vi "Csengő.vi"() -> ()   [LabVIEW 2014]
doc: "Az alkalmazás képes egy iskolai csengõ szerepét betölteni, csengetés hangot lejátszva a szükséges idõpontokban, figyelembe véve az aktuális tanév rendjét(ezt minden tanévben egyszer be kell állítani). Ezentúl beállítható, hogy a rendes, vagy a rövidített csengetési rend legyen érvényes egy adott napon. A szoftverben továbbá beállíthatóak olyan napok, mikor csak az elsõ n óra van megtartva. Segítségével egyszerûen, olcsón, az iskolarádióval egybevonva üzemeltethetõ az iskolacsengõ. A szoftver ezek mellett tûzriadó és bombariadó esetén képes riadójelzést sugározni.\n\nA mûködéssel kapcsolatos bõvebb információkért nyissa meg az alkalmazáson belül is megnyitható, az alkalmazás saját \"Olvass el!\" fájlát."
uses:
  <vilib>/Utility/file.llb/Read From Spreadsheet File (string).vi
  <vilib>/Utility/file.llb/Write To Spreadsheet File (string).vi
panel:
  out "Tanítási nap":bool
  in  "Segítség":bool
  out "Speciális tanítás":bool
  in  "Leállítás":bool
  in  "Módosítás":bool
  out "Kevesebb tanóra":bool
  out "Jelzõcsengõ":bool
  out "Csengõ":bool
  out "Munkaszüneti nap/\nSzünet":bool
  out "Napi max\nÓraszám:":i32
  out "Csengetési rend":string[][](array[string])
  out "Szünetek":string[][](array[string])
  out "Rövidített óra led":bool
  in  "Rövidített óra":bool
  out "Bombariadó LED":bool
  out "Tûzriadó LED":bool
  in  "Bombariadó":bool
  in  "Tûzriadó":bool
  # "Manuális vezérlés:"
  # "Tantervek módosítása"
  # "Táblázatok:"
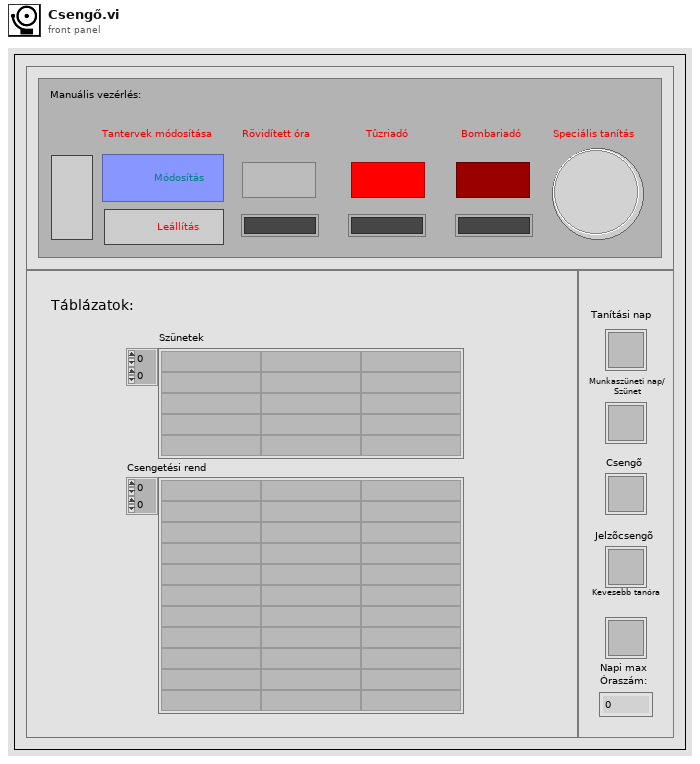
[diagram p1: front panel]
types:
  T1 = enum16{"open", "replace", "create", "open or create", "replace or create", "replace or create with confirmation"}
  T2 = typedef "LVDateTimeRec.ctl" = cluster{"fractional second":dbl, "second":i32, "minute":i32, "hour":i32, "day of month":i32, "month":i32, "year":i32, "day of week":i32, "day of year":i32, "DST":i32}
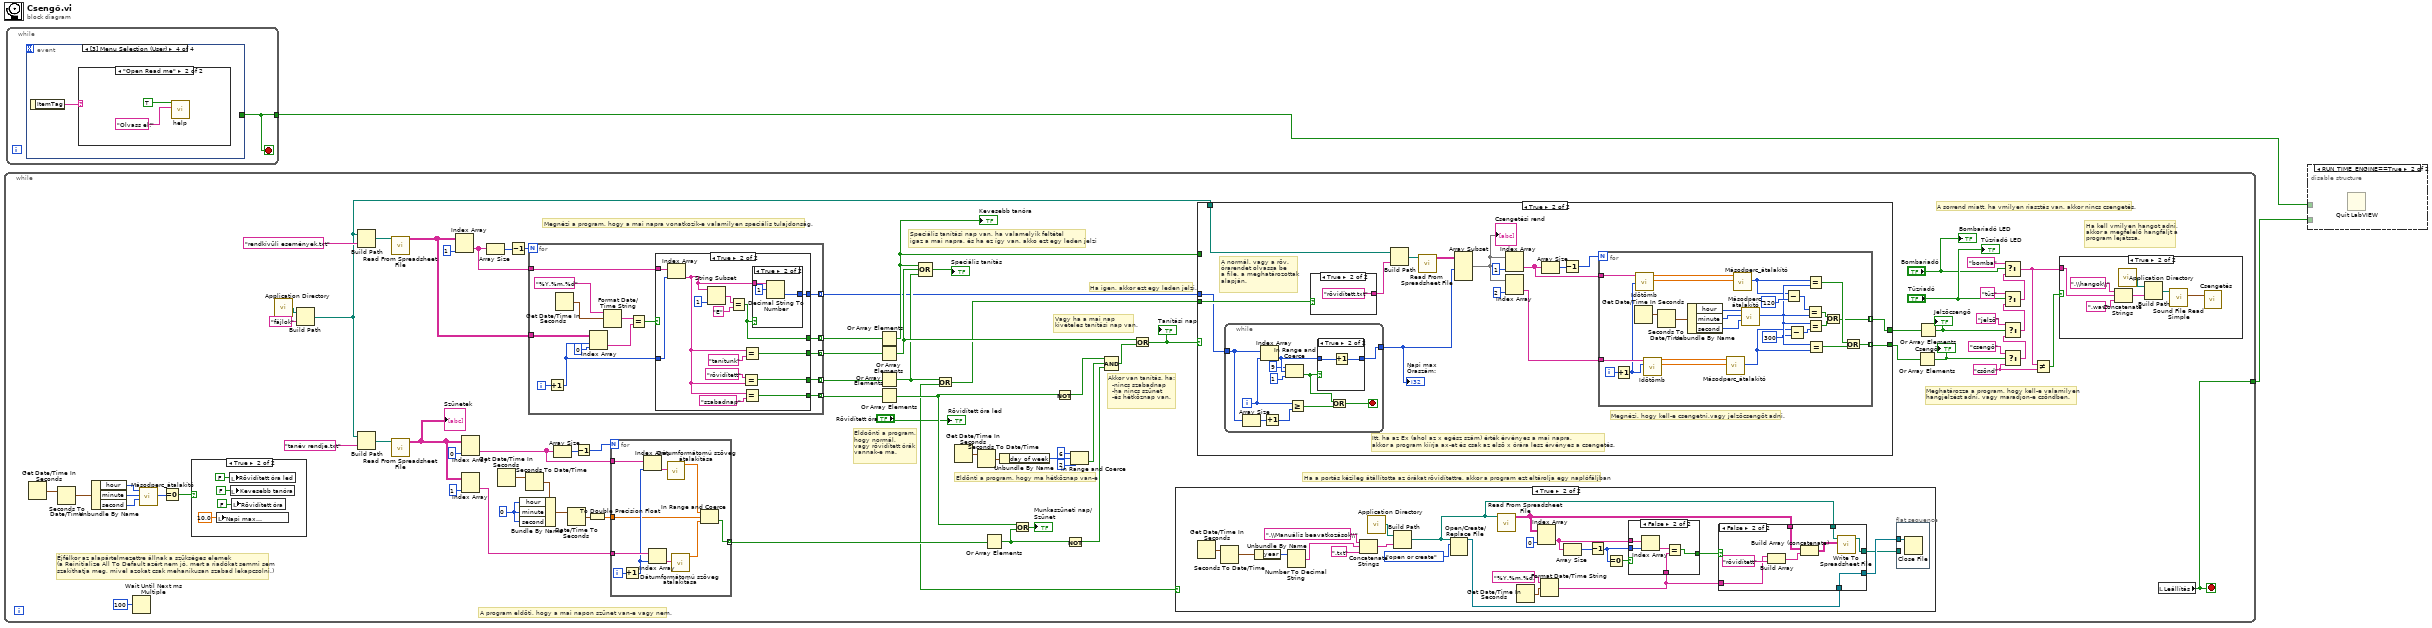
[diagram p0: block diagram]
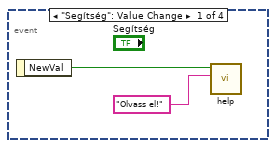
[diagram p3: hidden frame]
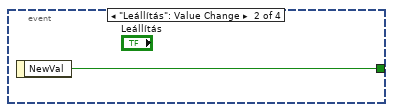
[diagram p4: hidden frame]
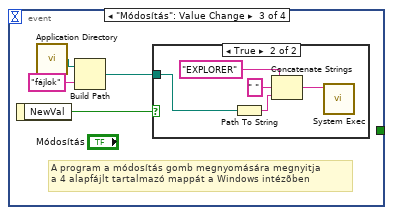
[diagram p5: hidden frame]
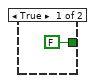
[diagram p11: hidden frame]
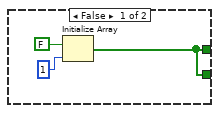
[diagram p13: hidden frame]
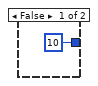
[diagram p14: hidden frame]
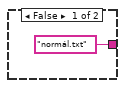
[diagram p15: hidden frame]
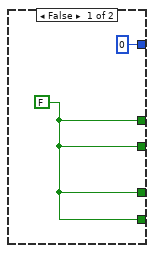
[diagram p16: hidden frame]
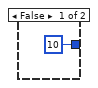
[diagram p17: hidden frame]
diagram:
  n1 = while {
    tunnel: [w3] -> w2
    stop <- w3 stop-if-true
    w36 = "csönd" ("format string")
    w61 = 0 ("hour")
    # "A sorrend miatt, ha vmilyen riasztás van, akkor nincs csengetés."
    # "Ha kell vmilyen hangot adni,\nakkor a megfelelõ hangfáljt a\nprogram lejátsza."
    # "Meghatározza a program, hogy kell-e valamilyen\nhangjelzést adni, vagy maradjon-e csöndben."
    # "Eldoönti a program,\nhogy normál,\nvagy rövidített órák\nvannak-e ma."
    # "Speciális tanítási nap van, ha valamelyik feltétel\nigaz a mai napra, és ha ez így van, akko ezt egy leden jelzi"
    # "Ha igen, akkor ezt egy leden jelzi."
    # "Eldönti a program, hogy ma hétköznap van-e"
    # "Vagy ha a mai nap\nkivételes tanítási nap van."
    # "Akkor van tanítás, ha:\n  -nincs szabadnap\n  -ha nincs szünet\n  -és hétköznap van."
    # "A program eldöti, hogy a mai napon szünet van-e vagy nem."
    # "Megnézi a program, hogy a mai napra vonatkozik-e valamilyen speciális tulajdonság."
    # "Ha a portás kézileg átállította az órákat rövidítettre, akkor a program ezt eltárolja egy naplófáljban"
    # "Éjfélkor az alapártelmezettre állnak a szükséges elemek\n(a Reinitialize All To Default azért nem jó, mert a riadókat semmi sem\nszakíthatja meg, mivel azokat csak mehanikusan szabad lekapcsolni.)"
    n2 = Get Date/Time In Seconds() -> (seconds since 1Jan1904=w13:timestamp)
    n3 = Seconds To Date/Time(time stamp (now)=w13) -> (date time rec=w12:T2)  [unwired: 1 in]
    n4 = Unbundle By Name(w12) -> ("hour"=w11:i32, "minute"=w10:i32, "second"=w9:i32)
    n5 = Wait Until Next ms Multiple(millisecond multiple=u32 100) -> ()  [unwired: 1 out]
    n6 = call "Másodperc_átalakító.vi"("Másodperc érték"=w9, "Perc érték"=w10, "Óra érték"=w11) -> ("Az összes érték másodpercben"=w14:i32)  [unwired: 8 in]
    n7 = Equal To 0?(x=w14) -> (x = 0?=w8:bool)
    n8 = case shown="True" w8 {
      frame False {
      }
      frame True {
        n9 = local write "Napi max\nÓraszám:"(10.0 ("Óraszám:")) -> ()
        n10 = local write "Rövidített óra led"(FALSE ("Rövidített óra led")) -> ()
        n11 = local write "Kevesebb tanóra"(FALSE ("Kevesebb tanóra")) -> ()
        n12 = local write "Rövidített óra"(FALSE ("Rövidített óra")) -> ()
      }
    }
    n13 = call <vilib>:"Application Directory.vi"() -> ("Application Directory"=w77:path)
    n14 = Build Path(base path=w77, name or relative path="fájlok") -> (appended path=w7:path)
    n15 = Build Path(base path=w7, name or relative path="rendkívüli események.txt") -> (appended path=w71:path)
    n16 = Build Path(base path=w7, name or relative path="tanév rendje.txt") -> (appended path=w69:path)
    n17 = call-poly <vilib>:"Read From Spreadsheet File.vi"("file path (dialog if empty)"=w71) -> ("all rows"=w49:string[][])  [unwired: 6 in, 4 out]
    n18 = call-poly <vilib>:"Read From Spreadsheet File.vi"("file path (dialog if empty)"=w69) -> ("all rows"=w41:string[][])  [unwired: 6 in, 4 out]
    "Szünetek" <- w41
    n19 = Index Array(array=w49, index (col)=1 ("index (row)")) -> (element=w50:string[])  [unwired: 1 in]
    n20 = Index Array(array=w41, index (col)=0 ("disabled index (col)")) -> (element=w57:string[])  [unwired: 1 in]
    n21 = Index Array(array=w41, index (col)=1 ("disabled index (col)")) -> (element=w53:string[])  [unwired: 1 in]
    n22 = Array Size(array=w50) -> (size(s)=w74:i32)
    n23 = Get Date/Time In Seconds() -> (seconds since 1Jan1904=w63:timestamp)
    n24 = Decrement(x=w74) -> (x-1=w72:i32)
    n25 = Seconds To Date/Time(time stamp (now)=w63) -> (date time rec=w62:T2)  [unwired: 1 in]
    n26 = Bundle By Name(cluster=w62, "hour"=w61, "minute"=w61, "second"=w61) -> (w60:T2)
    n27 = for {
      N: w72 -> [_]
      tunnel: w50 -> [w206]
      tunnel: w49 -> [w210]
      tunnel: [w204] -> w46 mode=indexing
      tunnel: [w203] -> w48 mode=indexing
      tunnel: [w202] -> w47 mode=indexing
      tunnel: [w201] -> w45 mode=indexing
      tunnel: [w200] -> w26 mode=indexing
      i -> [w214]
      n28 = Increment(x=w214) -> (x+1=w205:i32)
      n29 = Get Date/Time In Seconds() -> (seconds since 1Jan1904=w213:timestamp)
      n30 = Index Array(array=w210, index (row)=w205, index (col)=0 ("disabled index (col)")) -> (element=w208:string)
      n31 = Format Date/Time String(time format string (%c)="%Y.%m.%d" ("format string"), seconds (now)=w213) -> (date/time string=w211:string)  [unwired: 1 in]
      n32 = Equal?(x=w211, y=w208) -> (x = y?=w207:bool)
      n33 = case shown="True" w207 {
        tunnel: w206 -> [_ w230]
        tunnel: w205 -> [_ w229]
        tunnel: [w216 w225] -> w204
        tunnel: [w216 w224] -> w203
        tunnel: [w216 w223] -> w202
        tunnel: [w216 w219] -> w201
        tunnel: [0 w217] -> w200
        frame False {
          w216 = FALSE
        }
        frame True {
          n34 = Index Array(array=w230, index=w229) -> (element=w218:string)
          n35 = String Subset(string=w218, length (rest)=1 ("length (rest)")) -> (substring=w220:string)  [unwired: 1 in]
          n36 = Equal?(x=w220, y="E") -> (x = y?=w219:bool)
          n37 = Equal?(x="rövidített", y=w218) -> (x = y?=w224:bool)
          n38 = Equal?(x=w218, y="tanítunk" ("x")) -> (x = y?=w225:bool)
          n39 = Equal?(x=w218, y="szabadnap" ("x")) -> (x = y?=w223:bool)
          n40 = case shown="True" w219 {
            tunnel: w218 -> [_ w234]
            tunnel: [10 w232] -> w217
            frame False {
            }
            frame True {
              n41 = Decimal String To Number(string=w234, offset=1) -> (number=w232:i32)  [unwired: 1 in, 1 out]
            }
          }
        }
      }
    }
    n42 = Array Size(array=w57) -> (size(s)=w54:i32)
    n43 = Date/Time To Seconds(2:w60) -> (0:w59:timestamp)  [unwired: 1 in]
    n44 = Decrement(x=w54) -> (x-1=w55:i32)
    n45 = To Double Precision Float(number=w59) -> (double precision float=w52:dbl)
    n46 = for {
      N: w55 -> [_]
      tunnel: w57 -> [w199]
      tunnel: w53 -> [w197]
      tunnel: w52 -> [w193]
      tunnel: [w190] -> w51 mode=indexing
      i -> [w198]
      n47 = Increment(x=w198) -> (x+1=w196:i32)
      n48 = Index Array(array=w199, index=w196) -> (element=w194:string)
      n49 = Index Array(array=w197, index=w196) -> (element=w195:string)
      n50 = call "Dátumformátomú szöveg átalakítása.vi"("Szöveg, amiben keresni kell"=w194) -> ("Dátum értéke számban"=w191:dbl)  [unwired: 10 in]
      n51 = call "Dátumformátomú szöveg átalakítása.vi"("Szöveg, amiben keresni kell"=w195) -> ("Dátum értéke számban"=w192:dbl)  [unwired: 10 in]
      n52 = In Range and Coerce(upper limit=w191, x=w193, lower limit=w192) -> (In Range?=w190:bool)  [unwired: 1 out]
    }
    n53 = Or Array Elements(Boolean array=w45) -> (logical OR=w27:bool)
    "Kevesebb tanóra" <- w27
    n54 = Or Array Elements(Boolean array=w46) -> (logical OR=w44:bool)
    n55 = Or Array Elements(Boolean array=w48) -> (logical OR=w43:bool)
    n56 = Or Array Elements(Boolean array=w47) -> (logical OR=w16:bool)
    n57 = Compound Arithmetic op=OR(w27, w44, w43) -> (→"Speciális tanítás":bool)
    n58 = Or(x=w43, y="Rövidített óra") -> (x .or. y?=w42:bool)
    n59 = Get Date/Time In Seconds() -> (seconds since 1Jan1904=w64:timestamp)
    n60 = Seconds To Date/Time(time stamp (now)=w64) -> (date time rec=w65:T2)  [unwired: 1 in]
    n61 = Or Array Elements(Boolean array=w51) -> (logical OR=w17:bool)
    n62 = Unbundle By Name(w65) -> ("day of week"=w66:i32)
    n63 = Or(x=w16, y=w17) -> (x .or. y?=→"Munkaszüneti nap/\nSzünet":bool)
    n64 = Not(x=w16) -> (.not. x?=w18:bool)
    n65 = Not(x=w17) -> (.not. x?=w19:bool)
    n66 = In Range and Coerce(upper limit=6, x=w66, lower limit=2) -> (In Range?=w20:bool)  [unwired: 1 out]
    n67 = Compound Arithmetic op=AND(w18, w20, w19) -> (w22:bool)
    n68 = Or(x=w44, y=w22) -> (x .or. y?=w21:bool)
    "Tanítási nap" <- w21
    n69 = case shown="True" "Rövidített óra" {
      frame False {
      }
      frame True {
        n70 = Get Date/Time In Seconds() -> (seconds since 1Jan1904=w90:timestamp)
        n71 = Seconds To Date/Time(time stamp (now)=w90) -> (date time rec=w89:T2)  [unwired: 1 in]
        n72 = Unbundle By Name(w89) -> ("year"=w88:i32)
        n73 = Number To Decimal String(number=w88) -> (decimal integer string=w86:string)  [unwired: 1 in]
        n74 = Concatenate Strings(".\\Manuális beavatkozások\\" ("string"), w86, ".txt" ("string")) -> (w93:string)
        n75 = call <vilib>:"Application Directory.vi"() -> ("Application Directory"=w92:path)
        n76 = Build Path(base path=w92, name or relative path=w93) -> (appended path=w85:path)
        n77 = Open/Create/Replace File(file path (use dialog)=w85, operation (0:open)=T1."open or create") -> (refnum out=w83:refnum<file>)  [unwired: 4 in, 2 out]
        n78 = call-poly <vilib>:"Read From Spreadsheet File.vi"("file path (dialog if empty)"=w85) -> ("all rows"=w98:string[][])  [unwired: 6 in, 4 out]
        n79 = Get Date/Time In Seconds() -> (seconds since 1Jan1904=w104:timestamp)
        n80 = Index Array(array=w98, index (col)=0 ("disabled index (col)")) -> (element=w99:string[])  [unwired: 1 in]
        n81 = Format Date/Time String(time format string (%c)="%Y.%m.%d." ("format string"), seconds (now)=w104) -> (date/time string=w97:string)  [unwired: 1 in]
        n82 = Array Size(array=w99) -> (size(s)=w96:i32)
        n83 = Decrement(x=w96) -> (x-1=w95:i32)
        n84 = Equal To 0?(x=w95) -> (x = 0?=w101:bool)
        n85 = case shown="False" w101 {
          tunnel: w99 -> [_ w121]
          tunnel: w95 -> [_ w120]
          tunnel: w97 -> [_ w118]
          tunnel: [FALSE w117] -> w100
          frame True {
          }
          frame False {
            n86 = Index Array(array=w121, index=w120) -> (element=w119:string)
            n87 = Equal?(x=w119, y=w118) -> (x = y?=w117:bool)
          }
        }
        n88 = case shown="False" w100 {
          tunnel: w98 -> [_ w114]
          tunnel: w85 -> [w106 w111]
          tunnel: w97 -> [_ w110]
          tunnel: [w107 w109] -> w84
          tunnel: w83 -> [w107 w109]
          tunnel: [w106 w108] -> w82
          frame True {
          }
          frame False {
            n89 = Build Array(w110, "rövidített" ("x")) -> (w113:string[])
            n90 = Build Array (concatenate)(w114, w113) -> (w112:string[][])
            n91 = call-poly <vilib>:"Write To Spreadsheet File.vi"("2D data"=w112, "file path (dialog if empty)"=w111) -> ("new file path (Not A Path if cancelled)"=w108:path)  [unwired: 6 in]
          }
        }
        n92 = flat-sequence {
          tunnel: w84 -> [w105]
          tunnel: w82 -> [_]
          frame #0 {
            n93 = Close File(refnum=w105) -> ()  [unwired: 1 in, 2 out]
          }
        }
      }
    }
    n94 = case shown="True" w21 {
      tunnel: w7 -> [_ w133]
      tunnel: w42 -> [_ w139]
      tunnel: [w129 w138] -> w6
      tunnel: [w129 w134] -> w28
      tunnel: w27 -> [_ _]
      tunnel: w26 -> [_ w137]
      frame False {
        n95 = Initialize Array(FALSE, 1 ("dimension size")) -> (w129:bool[])
      }
      frame True {
        # "Megnézi, hogy kell-e csengetni,vagy jelzõcsengõt adni."
        # "A normál, vagy a röv.\nórarendet olvassa be\na file, a meghatározottak\nalapján."
        # "Itt, ha az Ex (ahol az x egész szám) érték érvényes a mai napra,\nakkor a program kiírja ax-et és csak az elsõ x órára lesz érvényes a csengetés."
        n96 = while {
          tunnel: w137 -> [w150]
          tunnel: [w154] -> w132
          i -> [w157]
          stop <- w151 stop-if-true
          n97 = Array Size(array=w150) -> (size(s)=w149:i32)
          n98 = Index Array(array=w150, index=w157) -> (element=w158:i32)
          n99 = Increment(x=w149) -> (x+1=w148:i32)
          n100 = In Range and Coerce(upper limit=9, x=w158, lower limit=1) -> (In Range?=w153:bool)  [unwired: 1 out]
          n101 = Greater Or Equal?(x=w157, y=w148) -> (x >= y?=w152:bool)
          n102 = case shown="True" w153 {
            tunnel: [10 w161] -> w154
            tunnel: w158 -> [_ w160]
            frame False {
            }
            frame True {
              n103 = Increment(x=w160) -> (x+1=w161:i32)
            }
          }
          n104 = Or(x=w153, y=w152) -> (x .or. y?=w151:bool)
        }
        "Napi max\nÓraszám:" <- w132
        n105 = case shown="True" w139 {
          tunnel: ["normál.txt" ("name or relative path") "rövidített.txt" ("name or relative path")] -> w140
          frame False {
          }
          frame True {
          }
        }
        n106 = Build Path(base path=w133, name or relative path=w140) -> (appended path=w141:path)
        n107 = call-poly <vilib>:"Read From Spreadsheet File.vi"("file path (dialog if empty)"=w141) -> ("all rows"=w136:string[][])  [unwired: 6 in, 4 out]
        n108 = Array Subset(array=w136, length (row)=w132) -> (w135:string[][])  [unwired: 3 in]
        "Csengetési rend" <- w135
        n109 = Index Array(array=w135, index (col)=1 ("disabled index (col)")) -> (element=w143:string[])  [unwired: 1 in]
        n110 = Index Array(array=w135, index (col)=2 ("disabled index (col)")) -> (element=w147:string[])  [unwired: 1 in]
        n111 = Array Size(array=w143) -> (size(s)=w146:i32)
        n112 = Decrement(x=w146) -> (x-1=w145:i32)
        n113 = for {
          N: w145 -> [_]
          tunnel: w143 -> [w170]
          tunnel: w147 -> [w169]
          tunnel: [w176] -> w134 mode=indexing
          tunnel: [w175] -> w138 mode=indexing
          i -> [w189]
          n114 = Increment(x=w189) -> (x+1=w168:i32)
          n115 = Get Date/Time In Seconds() -> (seconds since 1Jan1904=w187:timestamp)
          n116 = call "Idõtömb.vi"("Index"=w168, "Bemeneti tömb"=w170) -> ("Perc"=w166:dbl, "Óra"=w167:dbl)  [unwired: 8 in]
          n117 = call "Idõtömb.vi"("Index"=w168, "Bemeneti tömb"=w169) -> ("Perc"=w165:dbl, "Óra"=w164:dbl)  [unwired: 8 in]
          n118 = Seconds To Date/Time(time stamp (now)=w187) -> (date time rec=w186:T2)  [unwired: 1 in]
          n119 = Unbundle By Name(w186) -> ("hour"=w183:i32, "minute"=w184:i32, "second"=w185:i32)
          n120 = call "Másodperc_átalakító.vi"("Perc érték"=w165, "Óra érték"=w164) -> ("Az összes érték másodpercben"=w172:i32)  [unwired: 9 in]
          n121 = call "Másodperc_átalakító.vi"("Perc érték"=w166, "Óra érték"=w167) -> ("Az összes érték másodpercben"=w181:i32)  [unwired: 9 in]
          n122 = call "Másodperc_átalakító.vi"("Másodperc érték"=w185, "Perc érték"=w184, "Óra érték"=w183) -> ("Az összes érték másodpercben"=w182:i32)  [unwired: 8 in]
          n123 = Subtract(x=w181, y=120 ("x")) -> (x-y=w173:i32)
          n124 = Subtract(x=w172, y=300 ("x")) -> (x-y=w174:i32)
          n125 = Equal?(x=w173, y=w182) -> (x = y?=w180:bool)
          n126 = Equal?(x=w181, y=w182) -> (x = y?=w178:bool)
          n127 = Equal?(x=w182, y=w174) -> (x = y?=w179:bool)
          n128 = Equal?(x=w182, y=w172) -> (x = y?=w177:bool)
          n129 = Or(x=w180, y=w179) -> (x .or. y?=w176:bool)
          n130 = Or(x=w178, y=w177) -> (x .or. y?=w175:bool)
        }
      }
    }
    n131 = Or Array Elements(Boolean array=w6) -> (logical OR=w39:bool)
    "Csengõ" <- w39
    n132 = Or Array Elements(Boolean array=w28) -> (logical OR=w40:bool)
    "Jelzõcsengõ" <- w40
    n133 = Select(t="csengõ" ("format string"), s=w39, f=w36) -> (s? t:f=w30:string)
    n134 = Select(t="jelzõ", s=w40, f=w30) -> (s? t:f=w32:string)
    n135 = Select(t="tûz", s="Tûzriadó", f=w32) -> (s? t:f=w34:string)
    n136 = Select(t="bomba", s="Bombariadó", f=w34) -> (s? t:f=w38:string)
    n137 = Not Equal?(x=w38, y=w36) -> (x != y?=w37:bool)
    n138 = case shown="True" w37 {
      tunnel: w38 -> [_ w124]
      frame False {
      }
      frame True {
        n139 = Concatenate Strings(".\\hangok\\" ("string"), w124, ".wav" ("string")) -> (w126:string)
        n140 = call <vilib>:"Application Directory.vi"() -> ("Application Directory"=w125:path)
        n141 = Build Path(base path=w125, name or relative path=w126) -> (appended path=w122:path)
        n142 = call <vilib>:"Sound File Read Simple.vi"("path"=w122) -> ("data"=w123:waveform(dbl)[])  [unwired: 7 in, 3 out]
        n143 = call "Csengetés"("Data"=w123) -> ()  [unwired: 18 in, 1 out]
      }
    }
    n144 = local read "Leállítás"() -> (w3:bool)
    "Rövidített óra led" <- "Rövidített óra"
    "Tûzriadó LED" <- "Tûzriadó"
    "Bombariadó LED" <- "Bombariadó"
  }
  n145 = while {
    tunnel: [w235] -> w1
    stop <- w235 stop-if-true
    n146 = event shown="[3] Menu Selection (User)" {
      selector: _ -> [_ _ _ _]
      dyn-events: _ -> [_ _ _ _]
      timeout: _ -> [_ _ _ _]
      tunnel: [_ w238 _ _] -> w235
      event "Segítség": Value Change {
        n147 = event-data() -> ("NewVal"=w236:bool)  [unwired: 1 in]
        n148 = call "help.vi"("a fájl neve(.txt nem kell)"="Olvass el!", "Segítség"=w236) -> ()  [unwired: 10 in]
      }
      event "Leállítás": Value Change {
        n149 = event-data() -> ("NewVal"=w238:bool)  [unwired: 1 in]
      }
      event "Módosítás": Value Change {
        # "A program a módosítás gomb megnyomására megnyitja\na 4 alapfájlt tartalmazó mappát a Windows intézõben"
        n150 = event-data() -> ("NewVal"=w239:bool)  [unwired: 1 in]
        n151 = call <vilib>:"Application Directory.vi"() -> ("Application Directory"=w241:path)
        n152 = Build Path(base path=w241, name or relative path="fájlok") -> (appended path=w240:path)
        n153 = case shown="True" w239 {
          tunnel: w240 -> [_ w243]
          frame False {
          }
          frame True {
            n154 = Path To String(path=w243) -> (string=w247:string)
            n155 = Concatenate Strings("EXPLORER" ("string"), " " ("string"), w247) -> (w244:string)
            n156 = call <vilib>:"System Exec.vi"("command line"=w244) -> ()  [unwired: 7 in, 4 out]
          }
        }
      }
      event Menu Selection (User) {
        n157 = event-data() -> ("ItemTag"=w248:string)  [unwired: 1 in]
        n158 = case shown="\"Open Read me\"" w248 {
          frame Default {
          }
          frame "Open Read me" {
            n159 = call "help.vi"("a fájl neve(.txt nem kell)"="Olvass el!", "Segítség"=TRUE) -> ()  [unwired: 10 in]
          }
        }
      }
    }
  }
  n160 = disable-structure shown="RUN_TIME_ENGINE==True" {
    disable-tunnel: w2 -> [_ _]
    disable-tunnel: w1 -> [_ _]
    frame condition #0 (active) {
    }
    frame condition #1 {
      n161 = Quit LabVIEW() -> ()  [unwired: 1 in]
    }
  }
